vi "LEP_RV_OpBoxGlobal.vi"() -> ()   [LabVIEW 2011]
panel:
  in  "Text":string
  in  "Current Value":i32
  in  "Max Value":i32
  out "Stop":bool
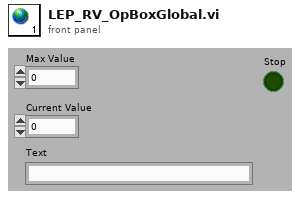
[diagram p1: front panel]
diagram:
